vi "Pade (x).vi"(0 "start":dbl, 5 "end":dbl, 7 "x":dbl, 9 "numerator":dbl[](array[numeric])=[0.0, 1.0, 0.0, -0.129957, 0.0, 0.0029035821005], 11 "denominator":dbl[](array[numeric])=[1.0, 0.0, 0.0367101138426, 0.0, 0.0006886010743, 0.0, 7.2619287682809e-06]) -> (4 "Pade (x)":dbl)   [LabVIEW 2025]
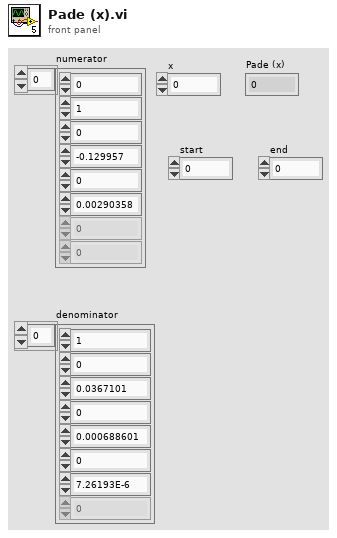
[diagram p1: front panel]
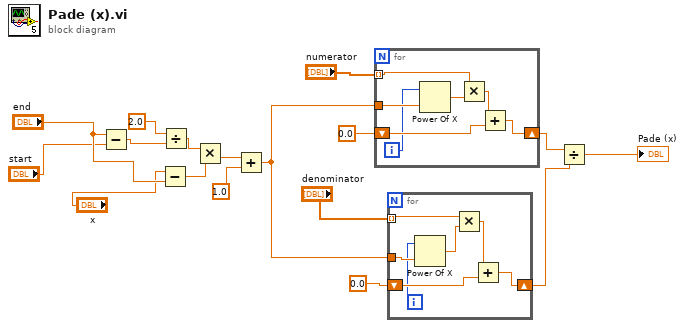
[diagram p0: block diagram]
diagram:
  n1 = Subtract(x="end", y="start") -> (x-y=w10:dbl)
  n2 = Subtract(x="x", y="end") -> (x-y=w7:dbl)
  n3 = Divide(x=2.0, y=w10) -> (x/y=w8:dbl)
  n4 = Multiply(x=w8, y=w7) -> (x*y=w6:dbl)
  n5 = Add(x=w6, y=1.0) -> (x+y=w2:dbl)
  n6 = for {
    tunnel: w2 -> [w24]
    tunnel: "numerator" -> [w20] mode=indexing
    shift-right: [w23] -> w16
    shift-left: 0.0 -> [w22]
    i -> [w18]
    n7 = Power Of X(1:w24, 2:w18) -> (0:w21:dbl)
    n8 = Multiply(x=w20, y=w21) -> (x*y=w19:dbl)
    n9 = Add(x=w19, y=w22) -> (x+y=w23:dbl)
  }
  n10 = for {
    tunnel: w2 -> [w31]
    tunnel: "denominator" -> [w28] mode=indexing
    shift-right: [w30] -> w17
    shift-left: 0.0 -> [w29]
    i -> [w25]
    n11 = Power Of X(1:w31, 2:w25) -> (0:w27:dbl)
    n12 = Multiply(x=w28, y=w27) -> (x*y=w26:dbl)
    n13 = Add(x=w26, y=w29) -> (x+y=w30:dbl)
  }
  n14 = Divide(x=w16, y=w17) -> (x/y=→"Pade (x)":dbl)
